vi "ImageAdapter.vi"(8 "error in (no error)":errorcluster, 10 "2D Picture":picture, 11 "Image in":T1) -> (0 "error out":errorcluster, 3 "Image Out":T1)   [LabVIEW 2012]
uses:
  <vilib>/vision/Image Controls.llb/IMAQ Image.ctl
  <vilib>/vision/NI_Vision_Development_Module.lvlib
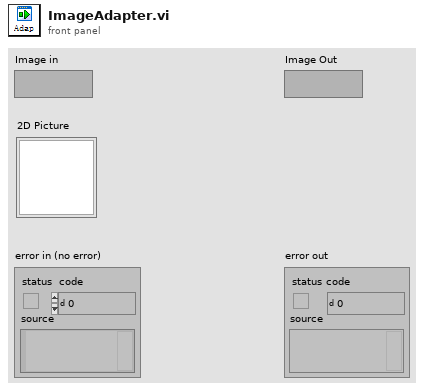
[diagram p1: front panel]
types:
  T1 = typedef "IMAQ Image.ctl" = refnum<image>
  T2 = typedef "Image Type" = u32
  T3 = typedef "imagedata.ctl" = cluster{"image type":i32, "image depth":i32, "image":u8[], "mask":u8[], "colors":u32[], "Rectangle":cluster{"left":i16, "top":i16, "right":i16, "bottom":i16}}
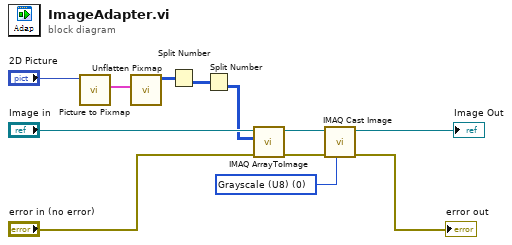
[diagram p0: block diagram]
diagram:
  w1 = T2 0 items=["Grayscale (U8)", "Grayscale (I16)", "Grayscale (SGL)", "Complex (CSG)", "RGB (U32)", "HSL (U32)", "RGB (U64)", "Grayscale (U16)"] ("Image Type")
  n1 = call <vilib>:"Picture to Pixmap.vi"("picture"="2D Picture") -> ("image data"=w10:T3)  [unwired: 9 in, 1 out]
  n2 = call <vilib>:"Unflatten Pixmap.vi"("image data"=w10) -> ("24-bit pixmap"=w12:u32[][])  [unwired: 4 in, 6 out]
  n3 = Split Number(x=w12) -> (lo(x)=w9:u16[][])  [unwired: 1 out]
  n4 = Split Number(x=w9) -> (lo(x)=w6:u8[][])  [unwired: 1 out]
  n5 = call "IMAQ ArrayToImage"("error in (no error)"="error in (no error)", "Image Pixels (U8)"=w6, "Image"="Image in") -> ("error out"=w3:errorcluster, "Image Out"=w5:T1)  [unwired: 7 in]
  n6 = call "IMAQ Cast Image"("Image Type"=w1, "error in (no error)"=w3, "Image Src"=w5) -> ("error out"=→"error out":errorcluster, "Image Dst Out"=→"Image Out":T1)  [unwired: 3 in, 4 out]
